vi "Read Functional Data.vi"   [LabVIEW 2016, in "Agilent E4980.lvlib"]
doc: "Reads AC Monitor, DC Monitor, Comparator BIN Count, Single Correction or Multiple Correction Data from the instrument."
uses:
  <instrlib>/Agilent E4980/Agilent E4980.lvlib
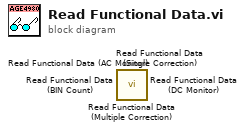
[diagram p0: block diagram]
diagram:
  n1 = call <instrlib>:"Read Functional Data (Multiple Correction).vi"() -> ()  [unwired: 9 in, 3 out]
  n2 = call <instrlib>:"Read Functional Data (Single Correction).vi"() -> ()  [unwired: 9 in, 3 out]
  n3 = call <instrlib>:"Read Functional Data (BIN Count).vi"() -> ()  [unwired: 9 in, 3 out]
  n4 = call <instrlib>:"Read Functional Data (DC Monitor).vi"() -> ()  [unwired: 8 in, 4 out]
  n5 = call <instrlib>:"Read Functional Data (AC Monitor).vi"() -> ()  [unwired: 8 in, 4 out]
